vi "GE 5565PIORC.DMA.Wait for Done Interrupt.vi"(8 "error in (no error)":errorcluster, 10 "timeout ms (1000)":u32=1000, 11 "GE 5565PIORC in":refnum<class "GE 5565PIORC.lvclass">) -> (0 "error out":errorcluster, 2 "timed out?":bool, 3 "GE 5565PIORC out":refnum<class "GE 5565PIORC.lvclass">)   [LabVIEW 2016, in "GE 5565PIORC.lvclass"]
uses:
  GE 5565PIORC.lvclass
  GE 5565PIORC.lvclass/GE 5565PIORC.ctl
  <vilib>/Utility/error.llb/Clear Errors.vi
  Properties/Registers/GE 5565PIORC.Registers.Local Configuration.Read.vi
  Properties/Registers/GE 5565PIORC.Registers.Local Configuration.Read (U8).vi
  Properties/Registers/GE 5565PIORC.Registers.Local Configuration.Write.vi
  Properties/Registers/GE 5565PIORC.Registers.Local Configuration.Write (U8).vi
  GE 5565PIORC.Bit Manipulation.Set Bit.vi
  GE 5565PIORC.Bit Manipulation.Set Bit (U8).vi
  GE 5565PIORC.Registers.Read.vi
  GE 5565PIORC.Registers.Read (U8).vi
  GE 5565PIORC.Registers.Write.vi
  GE 5565PIORC.Registers.Write (U8).vi
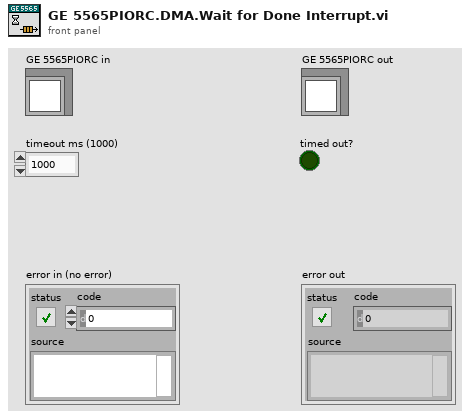
[diagram p1: front panel]
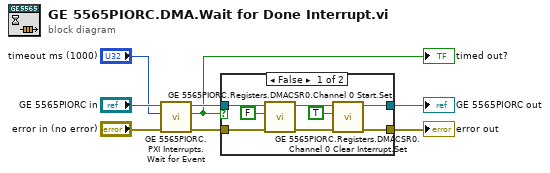
[diagram p0: block diagram]
diagram:
  n1 = call "GE 5565PIORC.PXI Interrupts.Wait for Event.vi"("error in (no error)"="error in (no error)", "timeout ms (1000)"="timeout ms (1000)", "GE 5565PIORC in"="GE 5565PIORC in") -> ("error out"=w5:errorcluster, "timed out?"=w1:bool, "GE 5565PIORC out"=w4:refnum<class "GE 5565PIORC.lvclass">)  [unwired: 6 in]
  "timed out?" <- w1
  n2 = case shown="False" w1 {
    tunnel: w5 -> [w16 w17]
    tunnel: w4 -> [w15 w18]
    tunnel: [w10 w18] -> w3
    tunnel: [w9 w17] -> w2
    frame False {
      n3 = call "GE 5565PIORC.Registers.DMACSR0.Channel 0 Start.Set.vi"("error in (no error)"=w16, "Channel 0 Start"=FALSE, "GE 5565PIORC in"=w15) -> ("error out"=w12:errorcluster, "GE 5565PIORC out"=w13:refnum<class "GE 5565PIORC.lvclass">)  [unwired: 7 in]
      n4 = call "GE 5565PIORC.Registers.DMACSR0.Channel 0 Clear Interrupt.Set.vi"("error in (no error)"=w12, "Channel 0 Clear Interrupt"=TRUE, "GE 5565PIORC in"=w13) -> ("error out"=w9:errorcluster, "GE 5565PIORC out"=w10:refnum<class "GE 5565PIORC.lvclass">)  [unwired: 7 in]
    }
    frame True {
    }
  }
  "GE 5565PIORC out" <- w3
  "error out" <- w2
